vi "CompareArray.vi"(10 "Array2":string[](array[string]), 11 "Array1":string[](array[string])) -> (1 "共同":string[](array[string]), 2 "Main":string[](array[string]), 3 "Sub":string[](array[string]))   [LabVIEW 2015]
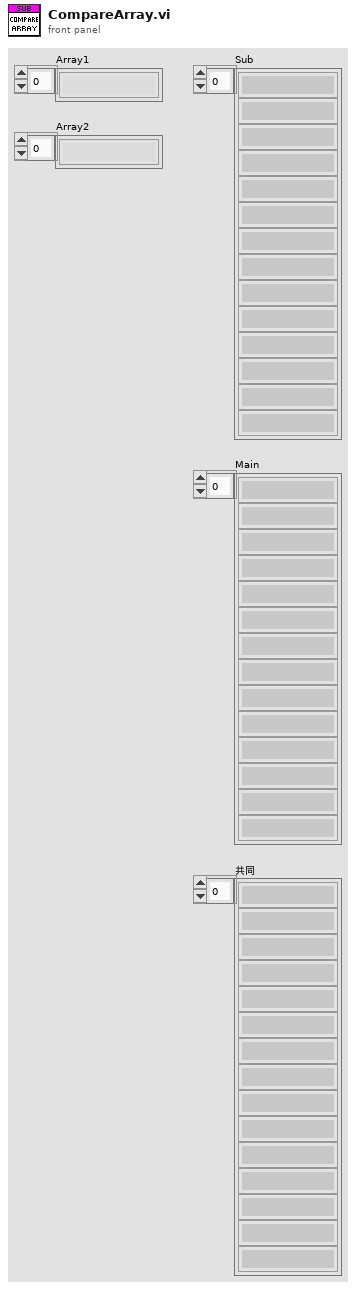
[diagram p1: front panel]
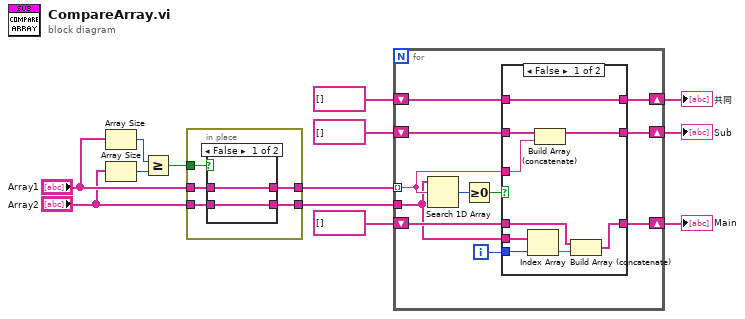
[diagram p0: block diagram]
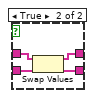
[diagram p2: hidden frame]
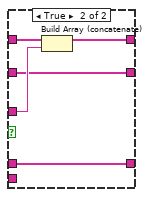
[diagram p3: hidden frame]
diagram:
  n1 = Array Size(array="Array1") -> (size(s)=w1:i32)
  n2 = Array Size(array="Array2") -> (size(s)=w2:i32)
  n3 = Greater Or Equal?(x=w1, y=w2) -> (x >= y?=w10:bool)
  n4 = in-place {
    in-place-border: "Array2" -> [w18]
    in-place-border: "Array1" -> [w17]
    in-place-border: [w16] -> w11
    in-place-border: [w15] -> w12
    in-place-border: w10 -> [w14]
    n5 = case shown="False" w14 {
      tunnel: w18 -> [w19 w24]
      tunnel: w17 -> [w20 w23]
      tunnel: [w20 w22] -> w16
      tunnel: [w19 w21] -> w15
      frame False {
      }
      frame True {
        n6 = Swap Values(12:w23, 14:w24) -> (1:w22:string[], 3:w21:string[])  [unwired: 1 in]
      }
    }
  }
  n7 = for {
    shift-right: [w33] -> w4
    shift-left: string[] [] -> [w34]
    tunnel: w12 -> [w29]
    tunnel: w11 -> [w32] mode=indexing
    shift-right: [w27] -> w8
    shift-left: string[] [] -> [w31]
    shift-right: [w28] -> w7
    shift-left: string[] [] -> [w30]
    i -> [w25]
    n8 = Search 1D Array(1D array=w29, element=w32) -> (index of element=w26:i32)  [unwired: 1 in]
    n9 = Greater Or Equal To 0?(x=w26) -> (x >= 0?=w35:bool)
    n10 = case shown="False" w35 {
      tunnel: [w44 w49] -> w33
      tunnel: w34 -> [w44 w48]
      tunnel: w32 -> [w42 w47]
      tunnel: w31 -> [w43 w46]
      tunnel: w30 -> [w41 w45]
      tunnel: w29 -> [w40 _]
      tunnel: [w39 w45] -> w28
      tunnel: [w38 w46] -> w27
      tunnel: w25 -> [w36 _]
      frame False {
        n11 = Index Array(array=w40, index=w36) -> (element=w37:string)
        n12 = Build Array (concatenate)(w43, w42) -> (w38:string[])
        n13 = Build Array (concatenate)(w41, w37) -> (w39:string[])
      }
      frame True {
        n14 = Build Array (concatenate)(w48, w47) -> (w49:string[])
      }
    }
  }
  "共同" <- w4
  "Main" <- w7
  "Sub" <- w8
